vi "Path String to Path Array.vi"(8 "error in (no error)":errorcluster, 11 "Path String":string) -> (0 "error out":errorcluster, 3 "Path Array":string[](array[string]))   [LabVIEW 2020, in "Variant Data Manipulation.lvlib"]
uses:
  Variant Data Manipulation.lvlib
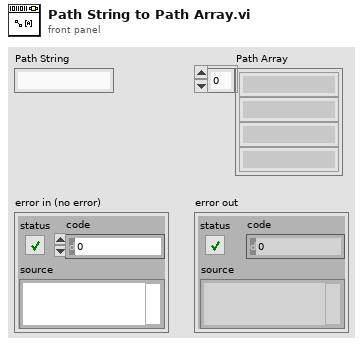
[diagram p1: front panel]
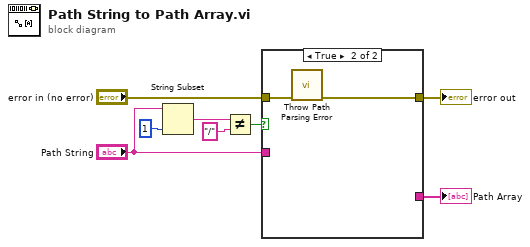
[diagram p0: block diagram]
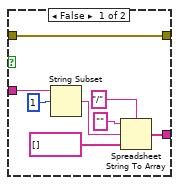
[diagram p2: hidden frame]
diagram:
  n1 = String Subset(string="Path String", length (rest)=1 ("length (rest)")) -> (substring=w6:string)  [unwired: 1 in]
  n2 = Not Equal?(x=w6, y="/") -> (x != y?=w4:bool)
  n3 = case shown="True" w4 {
    tunnel: "Path String" -> [w12 _]
    tunnel: [w13 w18] -> w3
    tunnel: "error in (no error)" -> [w13 w17]
    tunnel: [w9 _] -> w1
    frame False {
      n4 = String Subset(string=w12, offset (0)=1) -> (substring=w11:string)  [unwired: 1 in]
      n5 = Spreadsheet String To Array(delimiter (Tab)="/", format string="", spreadsheet string=w11, array type (2D Dbl)=string[] []) -> (array=w9:string[])
    }
    frame True {
      n6 = call "Throw Path Parsing Error.vi"("error in"=w17) -> ("error out"=w18:errorcluster)  [unwired: 10 in]
    }
  }
  "error out" <- w3
  "Path Array" <- w1
